vi "PSVCH_Formula Check.vi"(8 "Error In":errorcluster, 10 "VarList":cluster{"Tag":string[], "Alias":string[]}, 11 "Formula":string) -> (0 "Error Out":errorcluster, 1 "Formula Node out":T1, 2 "source":string, 3 "code":i32, 5 "VarList":T5)   [LabVIEW 2016]
uses:
  Ctrls/PSVCH_VarList.ctl
  ToolKit/Formula/Ctrls/PSFormula_FOR_Formula Node.ctl
  ToolKit/Formula/Ctrls/PSFormula_FOR_Formula Step.ctl
  ToolKit/Formula/Ctrls/PSFormula_FOR_Formula Para.ctl
  ToolKit/Formula/Ctrls/PSFormula_FOR_Formula MidVar Data.ctl
  Ctrls/PSVCH_Formula MidVar Data.ctl
  ToolKit/VARIANT Tool/Ctrls/PSVARIANT_Variant Para.ctl
  ToolKit/VARIANT Tool/Ctrls/PSVARIANT_Data Type.ctl
panel:
  # "Data Out"
  # "Data In"
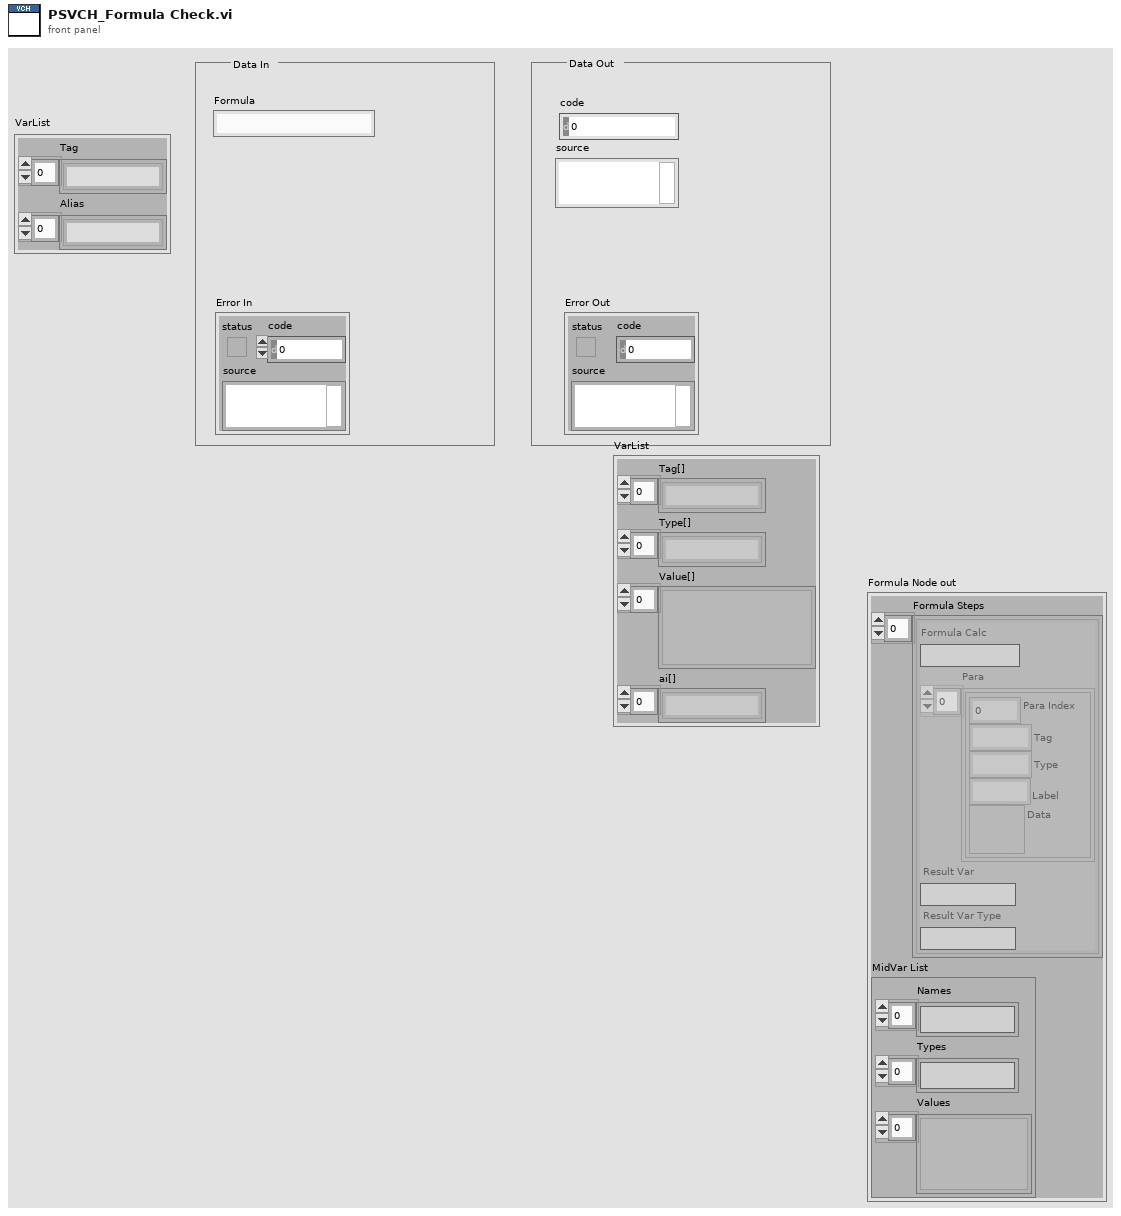
[diagram p1: front panel]
types:
  T1 = typedef "PSFormula_FOR_Formula Node.ctl" = cluster{"Formula Steps":T2[], "MidVar List":T4}
  T2 = typedef "PSFormula_FOR_Formula Step.ctl" = cluster{"Formula Calc":string, "Para":T3[], "Result Var":string, "Result Var Type":string}
  T3 = typedef "PSFormula_FOR_Formula Para.ctl" = cluster{"Para Index":i32, "Tag":string, "Type":string, "Label":string, "Data":variant}
  T4 = typedef "PSFormula_FOR_Formula MidVar Data.ctl" = cluster{"Names":string[], "Types":string[], "Values":variant[]}
  T5 = typedef "PSVCH_VarList.ctl" = cluster{"Tag[]":string[], "Type[]":string[], "Value[]":variant[], "ai[]":string[]}
  T6 = typedef "PSVCH_Formula MidVar Data.ctl" = cluster{"Names":string[], "Types":string[], "Values":variant[]}
  T7 = typedef "PSVARIANT_Variant Para.ctl" = cluster{"Label":string, "Type Data":T8[], "Type String":string, "Array Dimension":i32, "Variant":variant}
  T8 = typedef "PSVARIANT_Data Type.ctl" = u8
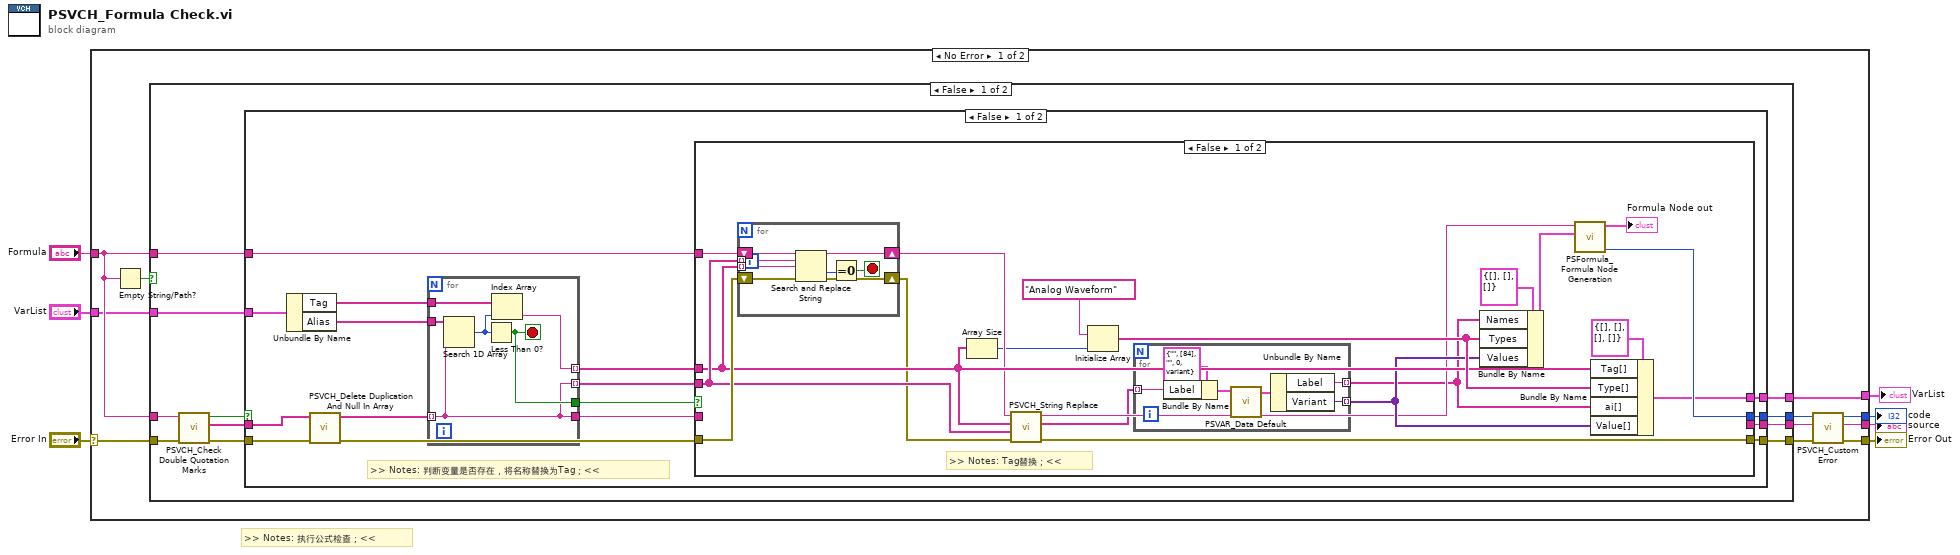
[diagram p0: block diagram]
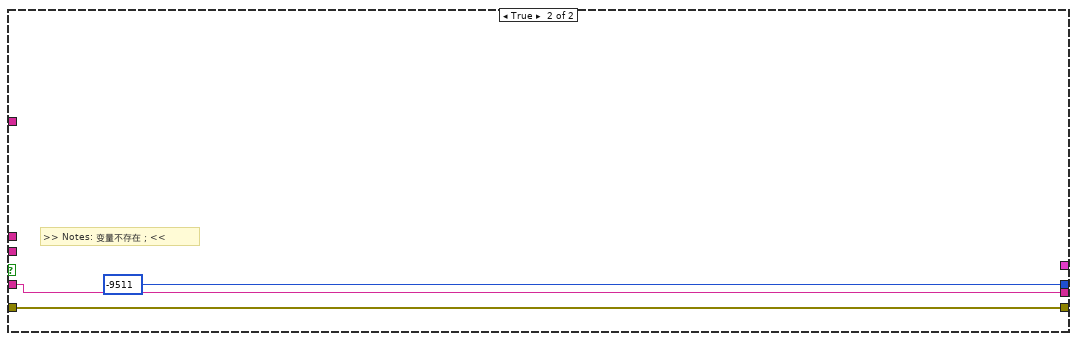
[diagram p2: hidden frame]
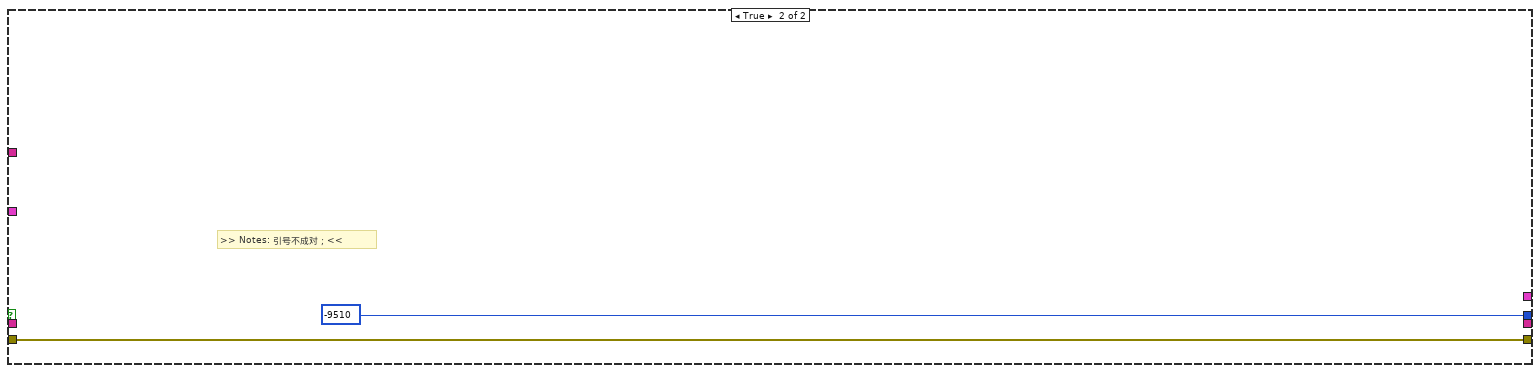
[diagram p3: hidden frame]
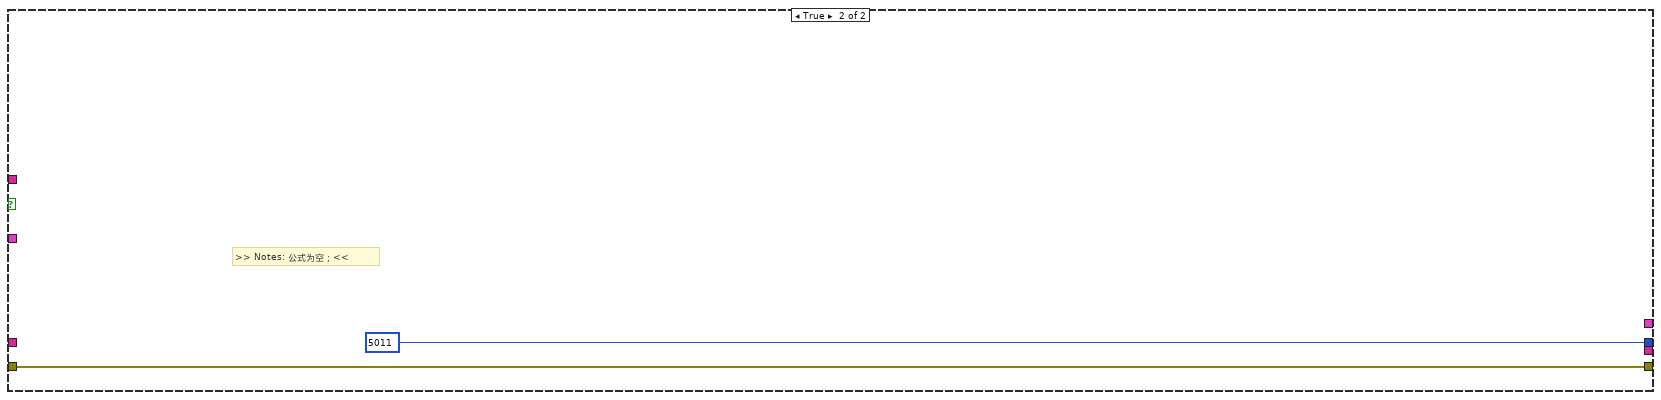
[diagram p4: hidden frame]
diagram:
  # ">> Notes: 执行公式检查；<<"
  n1 = case shown="No Error" "Error In" {
    selector: "Error In" -> [w17 w93]
    tunnel: [w14 w93] -> w5
    tunnel: "Formula" -> [w16 _]
    tunnel: [w13 _] -> w4
    tunnel: [w12 _] -> w3
    tunnel: "VarList" -> [w9 _]
    tunnel: [w8 _] -> w1
    frame No Error {
      n2 = Empty String/Path?(string/path=w16) -> (empty?=w18:bool)
      n3 = case shown="False" w18 {
        tunnel: w17 -> [w27 w91]
        tunnel: [w29 w91] -> w15
        tunnel: w16 -> [w23 _]
        tunnel: w16 -> [w28 _]
        tunnel: [w22 5011 ("Custom Code")] -> w11
        tunnel: [w21 _] -> w10
        tunnel: w9 -> [w20 _]
        tunnel: [w19 _] -> w8
        frame False {
          n4 = call "PSVCH_Check Double Quotation Marks.vi"("Error In (no error)"=w27, "String"=w23) -> ("Error Out"=w26:errorcluster, "\"Tag\"[]"=w25:string[], "Error?"=w24:bool)  [unwired: 7 in]
          n5 = case shown="False" w24 {
            tunnel: w26 -> [w37 w90]
            tunnel: [w42 w90] -> w29
            tunnel: w25 -> [w45 _]
            tunnel: w28 -> [w38 _]
            tunnel: [w35 -9510 ("Error Code")] -> w22
            tunnel: [w34 _] -> w21
            tunnel: w20 -> [w33 _]
            tunnel: [w30 _] -> w19
            frame False {
              # ">> Notes: 判断变量是否存在，将名称替换为Tag；<<"
              n6 = Unbundle By Name(w33) -> ("Tag"=w32:string[], "Alias"=w31:string[])
              n7 = call "PSVCH_Delete Duplication And Null In Array.vi"("Error In (no error)"=w37, "ArrayIn"=w45) -> ("Error Out"=w36:errorcluster, "ArrayOut"=w44:string[])  [unwired: 8 in]
              n8 = for {
                tunnel: w44 -> [w83] mode=indexing
                tunnel: w31 -> [w88]
                tunnel: [w83] -> w41
                tunnel: [w87] -> w43
                tunnel: w32 -> [w85]
                tunnel: [w84] -> w40 mode=indexing
                tunnel: [w83] -> w39 mode=indexing
                stop <- w87 stop-if-true
                n9 = Search 1D Array(1D array=w88, element=w83) -> (index of element=w86:i32)  [unwired: 1 in]
                n10 = Less Than 0?(x=w86) -> (x < 0?=w87:bool)
                n11 = Index Array(array=w85, index=w86) -> (element=w84:string)
              }
              n12 = case shown="False" w43 {
                tunnel: w36 -> [w57 w82]
                tunnel: [w65 w82] -> w42
                tunnel: w41 -> [_ w80]
                tunnel: w40 -> [w55 _]
                tunnel: w39 -> [w56 _]
                tunnel: w38 -> [w53 _]
                tunnel: [w62 -9511 ("Error Code")] -> w35
                tunnel: [_ w80] -> w34
                tunnel: [w58 _] -> w30
                frame False {
                  # ">> Notes: Tag替换；<<"
                  n13 = for {
                    shift-right: [w75] -> w52
                    shift-left: w53 -> [w79]
                    tunnel: w56 -> [w77] mode=indexing
                    tunnel: w55 -> [w76] mode=indexing
                    shift-right: [w72] -> w54
                    shift-left: w57 -> [w78]
                    stop <- w73 stop-if-true
                    n14 = Search and Replace String(input string=w79, search string=w77, replace string=w76, error in=w78) -> (result string=w75:string, offset past replacement=w74:i32, error out=w72:errorcluster)  [unwired: 4 in, 1 out]
                    n15 = Equal To 0?(x=w74) -> (x = 0?=w73:bool)
                  }
                  n16 = Array Size(array=w55) -> (size(s)=w51:i32)
                  n17 = call "PSVCH_String Replace.vi"("Error In (no error)"=w54, "ai[] In"=w56, "Tag[] In"=w55, "String In"=w52) -> ("Error Out"=w65:errorcluster, "ai[] Out"=w48:string[], "String Out"=w49:string)  [unwired: 4 in, 1 out]
                  n18 = Initialize Array("Analog Waveform", w51) -> (w59:string[])
                  n19 = for {
                    tunnel: [w68] -> w50 mode=indexing
                    tunnel: [w67] -> w46 mode=indexing
                    tunnel: w48 -> [w66] mode=indexing
                    n20 = Bundle By Name(cluster=T7 {"Label"="", "Type Data"=[84], "Type String"="", "Array Dimension"=0, "Variant"=variant} ("Data In"), "Label"=w66) -> (w70:T7)
                    n21 = call "PSVAR_Data Default.vi"("Data In"=w70) -> ("Data Default"=w69:T7)  [unwired: 9 in, 1 out]
                    n22 = Unbundle By Name(w69) -> ("Label"=w67:string, "Variant"=w68:variant)
                  }
                  n23 = Bundle By Name(cluster=T6 {"Names"=[], "Types"=[], "Values"=[]} ("Var List"), "Names"=w46, "Types"=w59, "Values"=w50) -> (w63:T6)
                  n24 = call "PSFormula_Formula Node Generation.vi"("Var List"=w63, "Fomula"=w49) -> ("Error Code"=w62:i32, "Formula Node"=→"Formula Node out":T1)  [unwired: 8 in]
                  n25 = Bundle By Name(cluster=T5 {"Tag[]"=[], "Type[]"=[], "Value[]"=[], "ai[]"=[]} ("输出簇"), "Tag[]"=w55, "Type[]"=w59, "ai[]"=w46, "Value[]"=w50) -> (w58:T5)
                }
                frame True {
                  # ">> Notes: 变量不存在；<<"
                }
              }
            }
            frame True {
              # ">> Notes: 引号不成对；<<"
            }
          }
        }
        frame True {
          # ">> Notes: 公式为空；<<"
        }
      }
      n26 = call "PSVCH_Custom Error.vi"("error in (no error)"=w15, "Source"=w10, "Custom Code"=w11) -> ("error out"=w14:errorcluster, "Explanation"=w12:string, "Custom Code"=w13:i32)  [unwired: 6 in]
    }
    frame Error {
    }
  }
  "Error Out" <- w5
  "code" <- w4
  "source" <- w3
  "VarList" <- w1
